vi "Set Offset.vi"(8 "error in (no error)":errorcluster, 10 "offset":u32, 11 "Transfer Configuration in":refnum<class "Transfer Configuration.lvclass">) -> (0 "error out":errorcluster, 3 "Transfer Configuration out":refnum<class "Transfer Configuration.lvclass">)   [LabVIEW 2020, in "GE Reflective Memory.lvlib" / "Transfer Configuration.lvclass"]
uses:
  Transfer Configuration.lvclass
  Transfer Configuration.lvclass/Transfer Configuration.ctl
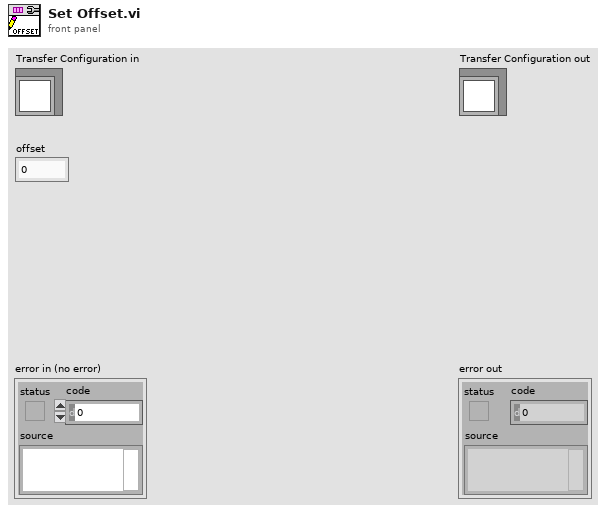
[diagram p1: front panel]
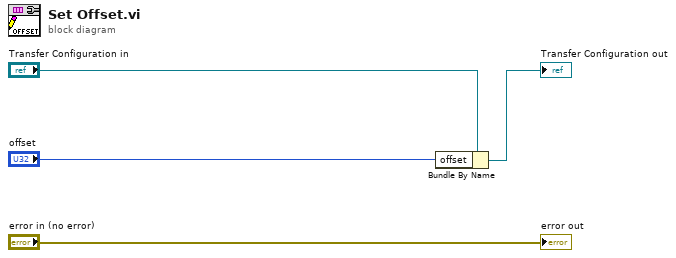
[diagram p0: block diagram]
diagram:
  n1 = Bundle By Name(cluster="Transfer Configuration in", "offset"="offset") -> (→"Transfer Configuration out":refnum<class "Transfer Configuration.lvclass">)
  "error out" <- "error in (no error)"
